vi "random_string.vi"(2 "length":i32=16) -> (7 "random string":string)   [LabVIEW 2015]
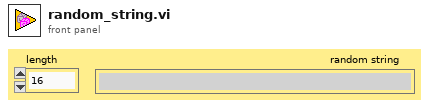
[diagram p1: front panel]
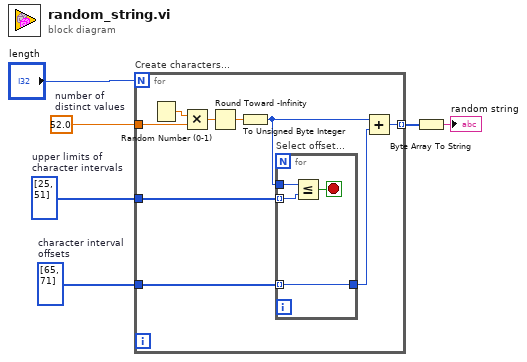
[diagram p0: block diagram]
diagram:
  w3 = u8[] [65, 71]  # character interval offsets
  w4 = u8[] [25, 51]  # upper limits of character intervals
  w6 = 52.0  # number of distinct values
  n1 = for "Create characters..." {
    N: "length" -> [_]
    tunnel: w6 -> [w15]
    tunnel: w4 -> [w11]
    tunnel: w3 -> [w10]
    tunnel: [w8] -> w5 mode=indexing
    n2 = Random Number (0-1)() -> (number: 0 to 1=w14:dbl)
    n3 = Multiply(x=w14, y=w15) -> (x*y=w13:dbl)
    n4 = Round Toward -Infinity(1:w13) -> (0:w12:dbl)
    n5 = To Unsigned Byte Integer(number=w12) -> (unsigned 8bit integer=w7:u8)
    n6 = for "Select offset..." {
      tunnel: w11 -> [w18] mode=indexing
      tunnel: w7 -> [w19]
      tunnel: w10 -> [w16] mode=indexing
      tunnel: [w16] -> w9
      stop <- w17 stop-if-true
      n7 = Less Or Equal?(x=w19, y=w18) -> (x <= y?=w17:bool)
    }
    n8 = Add(x=w7, y=w9) -> (x+y=w8:u8)
  }
  n9 = Byte Array To String(unsigned byte array=w5) -> (string=→"random string":string)
